vi "PRL Check Bad dt.vi"(11 "Allowed Increment":u64) -> (3 "Bad dt":bool)   [LabVIEW 2013, in "PMU Recorder Light.lvlib"]
doc: "Checks how many bad dt's have been detected since the last time this function was called."
uses:
  PMU Recorder Light.lvlib
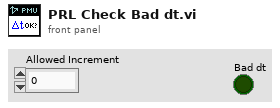
[diagram p1: front panel]
types:
  T1 = enum16{"Run", "Startup", "Get Status", "Pause", "Continue", "Shutdown", "Abort", "Open Panel", "Close Panel"}
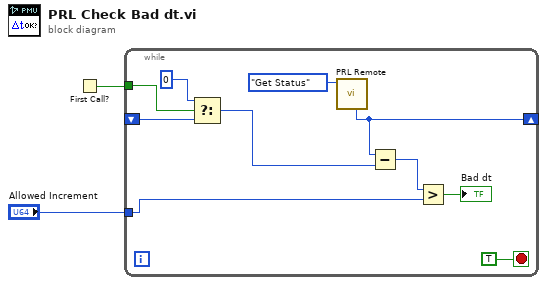
[diagram p0: block diagram]
diagram:
  n1 = First Call?() -> (First Call?: T/F=w2:bool)
  n2 = while {
    tunnel: w2 -> [w10]
    shift-right: [w8] -> _
    shift-left: _ -> [w9]
    tunnel: "Allowed Increment" -> [w5]
    stop <- TRUE stop-if-true
    n3 = Select(t=u64 0 ("Number of bad dt"), s=w10, f=w9) -> (s? t:f=w7:u64)
    n4 = call "PRL Remote.vi"("Action"=T1."Get Status") -> ("Number of bad dt"=w8:u64)  [unwired: 5 in, 5 out]
    n5 = Subtract(x=w8, y=w7) -> (x-y=w6:u64)
    n6 = Greater?(x=w6, y=w5) -> (0:→"Bad dt":bool)
  }
